vi "Normal User Default Chart holder FGV.vi"(1 "Action(GET)":T3(ring), 7 "Mem Ctl In":T1 {"LR2"."Line Width" items=["0", "1", "2", "3", "4", "5"]; "LR2"."Var Tag" items=["", "Wire Length", "Wire Tension", "Wire Speed", "Topside Voltage", "Tool Head Voltage", "Current", "Resistance"]; "LR1"."Line Width" items=["0", "1", "2", "3", "4", "5"]; "LR1"."Var Tag" items=["", "Wire Length", "Wire Tension", "Wire Speed", "Topside Voltage", "Tool Head Voltage", "Current", "Resistance"]; "LL2"."Line Width" items=["0", "1", "2", "3", "4", "5"]; "LL2"."Var Tag" items=["", "Wire Length", "Wire Tension", "Wire Speed", "Topside Voltage", "Tool Head Voltage", "Current", "Resistance"]; "LL1"."Line Width" items=["0", "1", "2", "3", "4", "5"]; "LL1"."Var Tag" items=["", "Wire Length", "Wire Tension", "Wire Speed", "Topside Voltage", "Tool Head Voltage", "Current", "Resistance"]; "UL1"."Line Width" items=["0", "1", "2", "3", "4", "5"]; "UL1"."Var Tag" items=["", "Wire Length", "Wire Tension", "Wire Speed", "Topside Voltage", "Tool Head Voltage", "Current", "Resistance"]; "UL2"."Line Width" items=["0", "1", "2", "3", "4", "5"]; "UL2"."Var Tag" items=["", "Wire Length", "Wire Tension", "Wire Speed", "Topside Voltage", "Tool Head Voltage", "Current", "Resistance"]; "UR2"."Line Width" items=["0", "1", "2", "3", "4", "5"]; "UR2"."Var Tag" items=["", "Wire Length", "Wire Tension", "Wire Speed", "Topside Voltage", "Tool Head Voltage", "Current", "Resistance"]; "UR1"."Line Width" items=["0", "1", "2", "3", "4", "5"]; "UR1"."Var Tag" items=["", "Wire Length", "Wire Tension", "Wire Speed", "Topside Voltage", "Tool Head Voltage", "Current", "Resistance"]}, 11 "error in (no error)":errorcluster) -> (8 "Mem Ctl Out":T1 {"LR2"."Line Width" items=["0", "1", "2", "3", "4", "5"]; "LR2"."Var Tag" items=["", "Wire Length", "Wire Tension", "Wire Speed", "Topside Voltage", "Tool Head Voltage", "Current", "Resistance"]; "LR1"."Line Width" items=["0", "1", "2", "3", "4", "5"]; "LR1"."Var Tag" items=["", "Wire Length", "Wire Tension", "Wire Speed", "Topside Voltage", "Tool Head Voltage", "Current", "Resistance"]; "LL2"."Line Width" items=["0", "1", "2", "3", "4", "5"]; "LL2"."Var Tag" items=["", "Wire Length", "Wire Tension", "Wire Speed", "Topside Voltage", "Tool Head Voltage", "Current", "Resistance"]; "LL1"."Line Width" items=["0", "1", "2", "3", "4", "5"]; "LL1"."Var Tag" items=["", "Wire Length", "Wire Tension", "Wire Speed", "Topside Voltage", "Tool Head Voltage", "Current", "Resistance"]; "UL1"."Line Width" items=["0", "1", "2", "3", "4", "5"]; "UL1"."Var Tag" items=["", "Wire Length", "Wire Tension", "Wire Speed", "Topside Voltage", "Tool Head Voltage", "Current", "Resistance"]; "UL2"."Line Width" items=["0", "1", "2", "3", "4", "5"]; "UL2"."Var Tag" items=["", "Wire Length", "Wire Tension", "Wire Speed", "Topside Voltage", "Tool Head Voltage", "Current", "Resistance"]; "UR2"."Line Width" items=["0", "1", "2", "3", "4", "5"]; "UR2"."Var Tag" items=["", "Wire Length", "Wire Tension", "Wire Speed", "Topside Voltage", "Tool Head Voltage", "Current", "Resistance"]; "UR1"."Line Width" items=["0", "1", "2", "3", "4", "5"]; "UR1"."Var Tag" items=["", "Wire Length", "Wire Tension", "Wire Speed", "Topside Voltage", "Tool Head Voltage", "Current", "Resistance"]}, 15 "error out":errorcluster)   [LabVIEW 2011]
uses:
  Graph default cluseter.ctl
  GUI/Graph/Plot selector.ctl
  <vilib>/Utility/VariantDataType/VariantType.lvlib
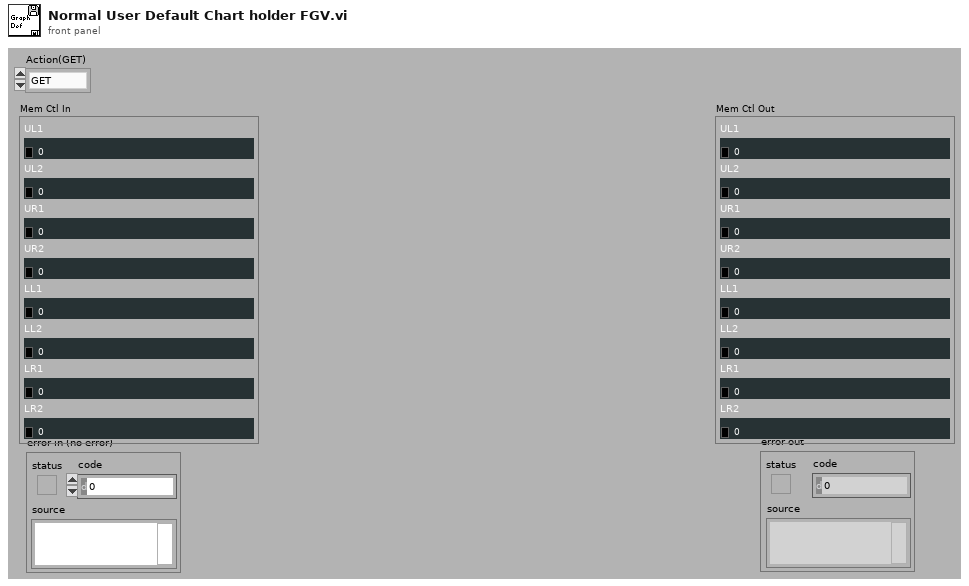
[diagram p1: front panel]
types:
  T1 = typedef "Graph default cluseter.ctl" = cluster{"UL1":T2, "UL2":T2, "UR1":T2, "UR2":T2, "LL1":T2, "LL2":T2, "LR1":T2, "LR2":T2}
  T2 = typedef "Plot selector.ctl" = cluster{"Var Tag":u16, "Color":u32, "Line Width":u16}
  T3 = enum16{"GET", "SET", "Get from Ini", "Put in Ini"}
  T4 = typedef "List of tools.ctl" = enum16{"Stroker", "Driller", "Tractor"}
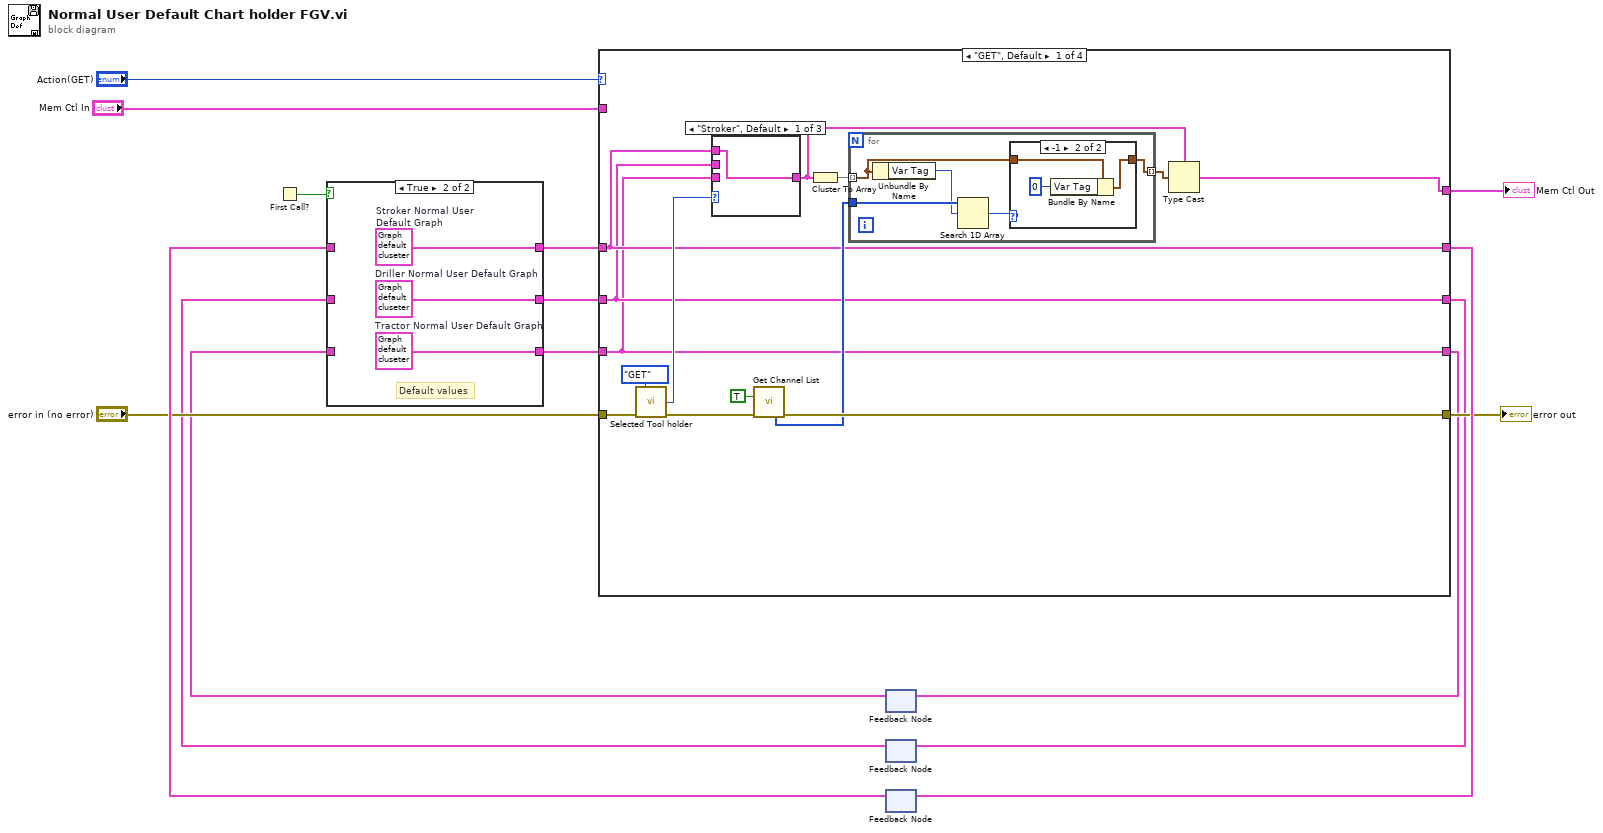
[diagram p0: block diagram]
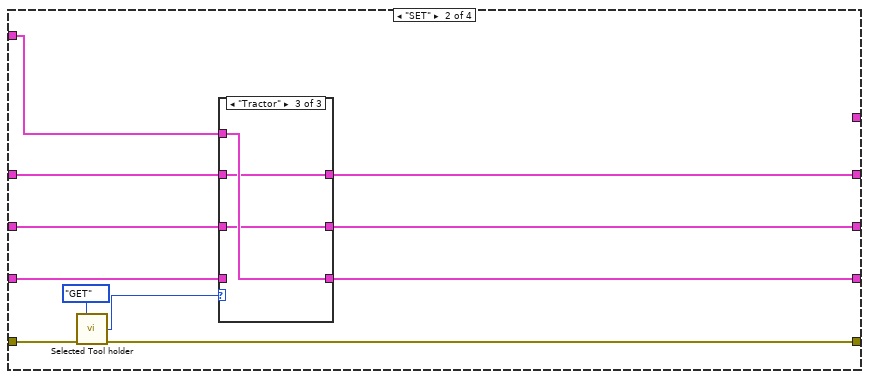
[diagram p6: hidden frame]
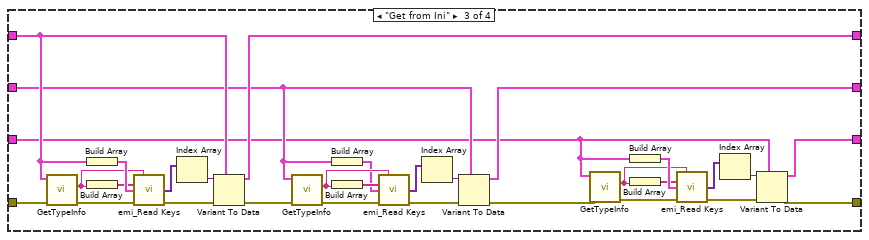
[diagram p9: hidden frame]
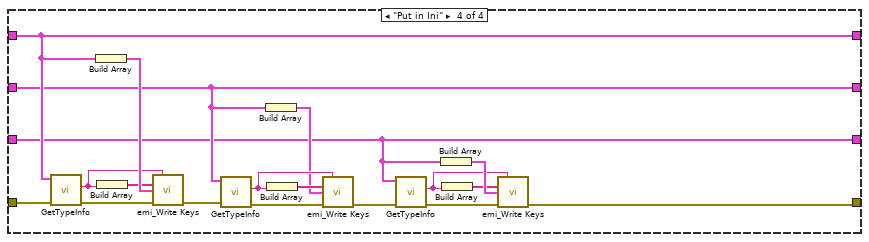
[diagram p10: hidden frame]
diagram:
  n1 = First Call?() -> (First Call?: T/F=w13:bool)
  n2 = feedback #1() -> (w4:T1)  [unwired: 1 in]
  n3 = feedback #2() -> (w5:T1)  [unwired: 1 in]
  n4 = feedback #3() -> (w14:T1)  [unwired: 1 in]
  n5 = case shown="True" w13 {
    tunnel: w14 -> [w18 _]
    tunnel: w5 -> [w17 _]
    tunnel: w4 -> [w16 _]
    tunnel: [w18 w21] -> w3
    tunnel: [w17 w20] -> w2
    tunnel: [w16 w19] -> w1
    frame False {
      (unwired) T1 {"UL1"={"Var Tag"=0, "Color"=0, "Line Width"=0}, "UL2"={"Var Tag"=0, "Color"=0, "Line Width"=0}, "UR1"={"Var Tag"=0, "Color"=0, "Line Width"=0}, "UR2"={"Var Tag"=0, "Color"=0, "Line Width"=0}, "LL1"={"Var Tag"=0, "Color"=0, "Line Width"=0}, "LL2"={"Var Tag"=0, "Color"=0, "Line Width"=0}, "LR1"={"Var Tag"=0, "Color"=0, "Line Width"=0}, "LR2"={"Var Tag"=0, "Color"=0, "Line Width"=0}}  # Normal User Default Graph
    }
    frame True {
      w19 = T1 {"UL1"={"Var Tag"=0, "Color"=16722194, "Line Width"=2}, "UL2"={"Var Tag"=0, "Color"=16771584, "Line Width"=2}, "UR1"={"Var Tag"=0, "Color"=1507583, "Line Width"=2}, "UR2"={"Var Tag"=0, "Color"=6618880, "Line Width"=2}, "LL1"={"Var Tag"=0, "Color"=16722194, "Line Width"=2}, "LL2"={"Var Tag"=0, "Color"=16771584, "Line Width"=2}, "LR1"={"Var Tag"=0, "Color"=1507583, "Line Width"=2}, "LR2"={"Var Tag"=0, "Color"=6618880, "Line Width"=2}}  # Tractor Normal User Default Graph
      w20 = T1 {"UL1"={"Var Tag"=0, "Color"=16722194, "Line Width"=2}, "UL2"={"Var Tag"=0, "Color"=16771584, "Line Width"=2}, "UR1"={"Var Tag"=0, "Color"=1507583, "Line Width"=2}, "UR2"={"Var Tag"=0, "Color"=6618880, "Line Width"=2}, "LL1"={"Var Tag"=0, "Color"=16722194, "Line Width"=2}, "LL2"={"Var Tag"=0, "Color"=16771584, "Line Width"=2}, "LR1"={"Var Tag"=0, "Color"=1507583, "Line Width"=2}, "LR2"={"Var Tag"=0, "Color"=6618880, "Line Width"=2}}  # Driller Normal User Default Graph
      w21 = T1 {"UL1"={"Var Tag"=0, "Color"=16722194, "Line Width"=2}, "UL2"={"Var Tag"=0, "Color"=16771584, "Line Width"=2}, "UR1"={"Var Tag"=0, "Color"=1507583, "Line Width"=2}, "UR2"={"Var Tag"=0, "Color"=6618880, "Line Width"=2}, "LL1"={"Var Tag"=0, "Color"=16722194, "Line Width"=2}, "LL2"={"Var Tag"=0, "Color"=16771584, "Line Width"=2}, "LR1"={"Var Tag"=0, "Color"=1507583, "Line Width"=2}, "LR2"={"Var Tag"=0, "Color"=6618880, "Line Width"=2}}  # Stroker Normal User Default Graph
      # "Default values"
    }
  }
  n6 = case shown="\"GET\", Default" "Action(GET)" {
    tunnel: [w26 w54 w89 w101] -> w12
    tunnel: "error in (no error)" -> [w27 w57 w98 w117]
    tunnel: [w35 w56 w69 w102] -> w10
    tunnel: [w34 _ _ _] -> w8
    tunnel: "Mem Ctl In" -> [_ w51 _ _]
    tunnel: [w25 w53 w72 w100] -> w6
    tunnel: [w24 w52 w68 w99] -> w7
    tunnel: w3 -> [w26 w50 w92 w101]
    tunnel: w2 -> [w25 w49 w71 w100]
    tunnel: w1 -> [w24 w48 w70 w99]
    frame "GET", Default {
      n7 = call "Selected Tool holder.vi"("Action(GET)"=enum16{"GET", "SET"}."GET", "error in (no error)"=w27) -> ("Tool out"=w28:T4, "error out"=w23:errorcluster)  [unwired: 12 in]
      n8 = case shown="\"Stroker\", Default" w28 {
        tunnel: w26 -> [w36 _ _]
        tunnel: w25 -> [_ w37 _]
        tunnel: w24 -> [_ _ w38]
        tunnel: [w36 w37 w38] -> w22
        frame "Stroker", Default {
        }
        frame "Driller" {
        }
        frame "Tractor" {
        }
      }
      n9 = call "Get Channel List.vi"("Force all(F)"=TRUE, "error in"=w23) -> ("Value list"=w33:u16[], "error out"=w35:errorcluster)  [unwired: 9 in, 3 out]
      n10 = Cluster To Array(cluster=w22) -> (array=w32:T2[])
      n11 = for {
        tunnel: [w39] -> w31 mode=indexing
        tunnel: w32 -> [w40] mode=indexing
        tunnel: w33 -> [w43]
        n12 = Unbundle By Name(w40) -> ("Var Tag"=w42:u16)
        n13 = Search 1D Array(1D array=w43, element=w42) -> (index of element=w41:i32)  [unwired: 1 in]
        n14 = case shown="-1" w41 {
          tunnel: w40 -> [w44 w47]
          tunnel: [w44 w46] -> w39
          frame 0, Default {
          }
          frame -1 {
            n15 = Bundle By Name(cluster=w47, "Var Tag"=u16 0) -> (w46:T2)
          }
        }
      }
      n16 = Type Cast(type=w22, x=w31) -> (*(type *) &x=w34:T1)
    }
    frame "SET" {
      n17 = call "Selected Tool holder.vi"("Action(GET)"=enum16{"GET", "SET"}."GET", "error in (no error)"=w57) -> ("Tool out"=w55:T4, "error out"=w56:errorcluster)  [unwired: 12 in]
      n18 = case shown="\"Tractor\"" w55 {
        tunnel: w51 -> [w61 w62 w67]
        tunnel: w48 -> [w59 w64 _]
        tunnel: w49 -> [w60 _ w66]
        tunnel: w50 -> [_ w63 w65]
        tunnel: [w60 w62 w66] -> w53
        tunnel: [w59 w64 w67] -> w52
        tunnel: [w61 w63 w65] -> w54
        frame "Stroker", Default {
        }
        frame "Driller" {
        }
        frame "Tractor" {
        }
      }
    }
    frame "Get from Ini" {
      n19 = call <vilib>:"GetTypeInfo.vi"("error in (no error)"=w98, "Variant"=w92) -> ("error out"=w94:errorcluster, "Name"=w93:string)  [unwired: 5 in, 3 out]
      n20 = Build Array(w92) -> (w97:T1[])
      n21 = Build Array(w93) -> (w96:string[])
      n22 = call "emi_Read Keys.vi"("Section"=w93, "Key Names"=w96, "Types/Defaults"=w97, "error in (no error)"=w94) -> ("Values"=w95:variant[], "error out"=w90:errorcluster)  [unwired: 9 in, 1 out]
      n23 = Index Array(array=w95) -> (element=w91:variant)  [unwired: 1 in]
      n24 = Variant To Data(error in=w90, type=w92, Variant=w91) -> (data=w89:T1, error out=w81:errorcluster)
      n25 = call <vilib>:"GetTypeInfo.vi"("error in (no error)"=w81, "Variant"=w71) -> ("error out"=w85:errorcluster, "Name"=w86:string)  [unwired: 5 in, 3 out]
      n26 = Build Array(w71) -> (w82:T1[])
      n27 = Build Array(w86) -> (w83:string[])
      n28 = call "emi_Read Keys.vi"("Section"=w86, "Key Names"=w83, "Types/Defaults"=w82, "error in (no error)"=w85) -> ("Values"=w84:variant[], "error out"=w88:errorcluster)  [unwired: 9 in, 1 out]
      n29 = Index Array(array=w84) -> (element=w87:variant)  [unwired: 1 in]
      n30 = Variant To Data(error in=w88, type=w71, Variant=w87) -> (data=w72:T1, error out=w73:errorcluster)
      n31 = call <vilib>:"GetTypeInfo.vi"("error in (no error)"=w73, "Variant"=w70) -> ("error out"=w77:errorcluster, "Name"=w76:string)  [unwired: 5 in, 3 out]
      n32 = Build Array(w70) -> (w80:T1[])
      n33 = Build Array(w76) -> (w79:string[])
      n34 = call "emi_Read Keys.vi"("Section"=w76, "Key Names"=w79, "Types/Defaults"=w80, "error in (no error)"=w77) -> ("Values"=w78:variant[], "error out"=w74:errorcluster)  [unwired: 9 in, 1 out]
      n35 = Index Array(array=w78) -> (element=w75:variant)  [unwired: 1 in]
      n36 = Variant To Data(error in=w74, type=w70, Variant=w75) -> (data=w68:T1, error out=w69:errorcluster)
    }
    frame "Put in Ini" {
      n37 = call <vilib>:"GetTypeInfo.vi"("error in (no error)"=w117, "Variant"=w101) -> ("error out"=w114:errorcluster, "Name"=w113:string)  [unwired: 5 in, 3 out]
      n38 = Build Array(w101) -> (w116:T1[])
      n39 = Build Array(w113) -> (w115:string[])
      n40 = call "emi_Write Keys.vi"("Section"=w113, "Key Names"=w115, "Values"=w116, "error in (no error)"=w114) -> ("error out"=w104:errorcluster)  [unwired: 10 in, 1 out]
      n41 = call <vilib>:"GetTypeInfo.vi"("error in (no error)"=w104, "Variant"=w100) -> ("error out"=w111:errorcluster, "Name"=w112:string)  [unwired: 5 in, 3 out]
      n42 = Build Array(w100) -> (w109:T1[])
      n43 = Build Array(w112) -> (w110:string[])
      n44 = call "emi_Write Keys.vi"("Section"=w112, "Key Names"=w110, "Values"=w109, "error in (no error)"=w111) -> ("error out"=w103:errorcluster)  [unwired: 10 in, 1 out]
      n45 = call <vilib>:"GetTypeInfo.vi"("error in (no error)"=w103, "Variant"=w99) -> ("error out"=w106:errorcluster, "Name"=w105:string)  [unwired: 5 in, 3 out]
      n46 = Build Array(w99) -> (w108:T1[])
      n47 = Build Array(w105) -> (w107:string[])
      n48 = call "emi_Write Keys.vi"("Section"=w105, "Key Names"=w107, "Values"=w108, "error in (no error)"=w106) -> ("error out"=w102:errorcluster)  [unwired: 10 in, 1 out]
    }
  }
  "error out" <- w10
  "Mem Ctl Out" <- w8
  n49 = feedback-in #1(w7) -> ()
  n50 = feedback-in #2(w6) -> ()
  n51 = feedback-in #3(w12) -> ()
